vi "ex5-8.vi"() -> ()   [LabVIEW 2014]
uses:
  <vilib>/NXT/Subs/MotorOutput.ctl
  <vilib>/NXT/Block Support/NXT_ButtonSelector.ctl
  <vilib>/NXT/Dual Mode Library/Sensors/readNXTButton.vi
  <vilib>/NXT/Dual Mode Library/Motors/MotorBrake.vi
panel:
  out "機器人舵向":sgl(graph)
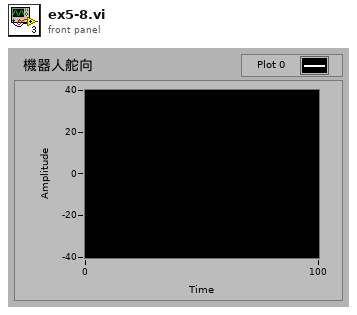
[diagram p1: front panel]
types:
  T1 = typedef "MotorOutput.ctl" = u8
  T2 = typedef "LVHSConnector.ctl" = refnum<class "BrickReference.lvclass">
  T3 = typedef "NXT_ButtonSelector.ctl" = u16
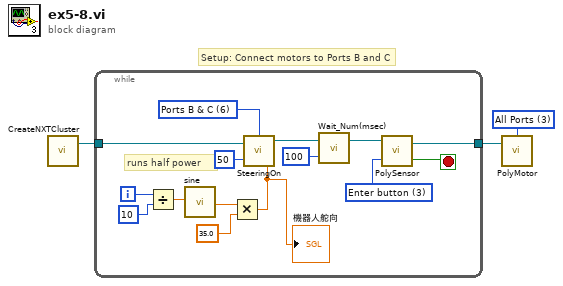
[diagram p0: block diagram]
diagram:
  w2 = T1 3 items=["Port A", "Port B", "Port C", "All Ports"] ("Output Port")
  # "Setup: Connect motors to Ports B and C"
  n1 = call <vilib>:"CreateNXTCluster.vi"() -> ("NXT/EV3"=w3:T2)  [unwired: 4 in]
  n2 = while {
    tunnel: w3 -> [w18]
    tunnel: [w17] -> w1
    i -> [w10]
    stop <- w16 stop-if-true
    w4 = T1 6 items=["Port A"=0, "Port B"=1, "Port C"=2, "Ports A & B"=4, "Ports A & C"=5, "Ports B & C"=6, "All Ports"=3] ("Output Ports (A & B)")
    w15 = T3 3 items=["Enter button"=3, "Left button"=2, "Right button"=1] ("Button (Enter button)")
    # "runs half power"
    n3 = Divide(x=w10, y=10 ("x")) -> (x/y=w12:dbl)
    n4 = call <vilib>:"sine.vi"("x"=w12) -> ("sin(x)"=w14:sgl)
    n5 = Multiply(x=w14, y=sgl 35.0) -> (x*y=w5:sgl)
    "機器人舵向" <- w5
    n6 = call <vilib>:"SteeringOn.vi"("Power (75)"=50, "Steering (100)"=w5, "NXT/EV3"=w18, "Output Ports (A & B)"=w4) -> ("NXT/EV3"=w8:T2)
    n7 = call <vilib>:"Wait_Num(msec).vi"("Time (100 msec)"=u32 100 ("Time (msec)"), "NXT/EV3"=w8) -> ("NXT/EV3"=w9:T2)  [unwired: 2 in]
    n8 = call-poly <vilib>:"PolySensor.vi"("Button (Enter button)"=w15, "NXT/EV3"=w9) -> ("Yes/No"=w16:bool, "NXT/EV3"=w17:T2)  [unwired: 1 out]
  }
  n9 = call-poly <vilib>:"PolyMotor.vi"("NXT/EV3"=w1, "Port (All Ports)"=w2) -> ()  [unwired: 3 out]
